vi "Settings Memory.vi"(6 "Write?":bool, 7 "Setting Choice":T2, 10 "Input":variant) -> (1 "PRL dt Tolerance":dbl, 2 "Output Int32":i32, 3 "Config Settings":T1)   [LabVIEW 2013, in "PMU Recorder Light.lvlib"]
uses:
  PMU Recorder Light.lvlib
  Configuration Settings.ctl
  Setting Choice.ctl
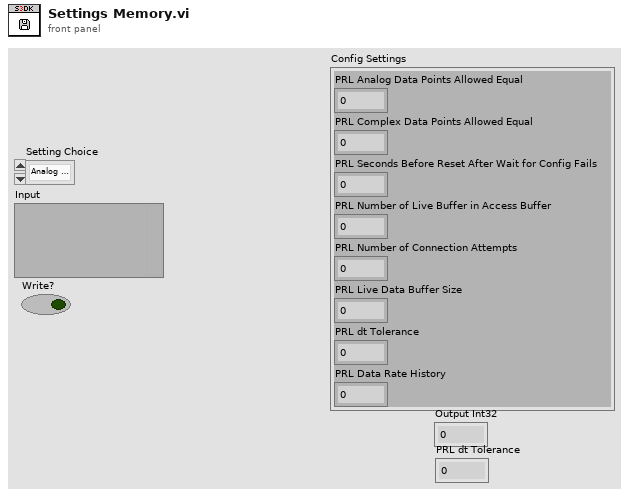
[diagram p1: front panel]
types:
  T1 = typedef "PMU Recorder Light.lvlib/Configuration Settings.ctl" = cluster{"PRL Analog Data Points Allowed Equal":i32, "PRL Complex Data Points Allowed Equal":i32, "PRL Seconds Before Reset After Wait for Config Fails":i32, "PRL Number of Live Buffer in Access Buffer":i32, "PRL Number of Connection Attempts":i32, "PRL Live Data Buffer Size":i32, "PRL dt Tolerance":dbl, "PRL Data Rate History":i32}
  T2 = typedef "PMU Recorder Light.lvlib/Setting Choice.ctl" = enum16{"Analog Data Points Allowed Equals", "Complex Data Points Allowed Equals", "Seconds Before Reset After Wait for Config Fails", "Number of Live Buffer in Access Buffer ", "Number of Connection Attempts", "Live Data Buffer Size", "dt Tolerance", "Data Rate History", "ALL"}
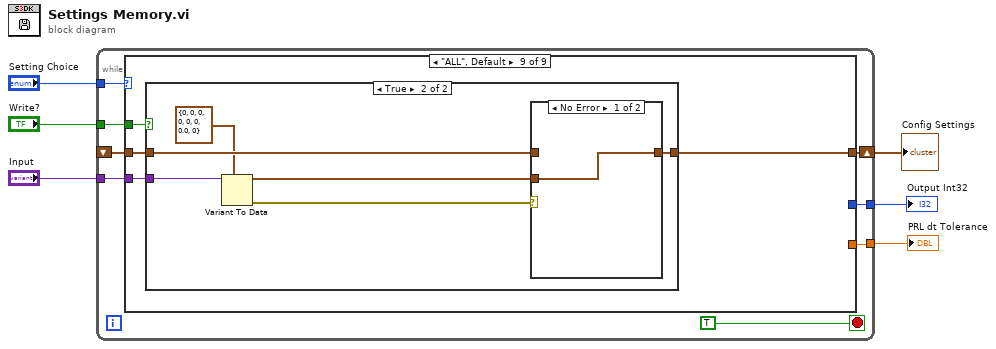
[diagram p0: block diagram]
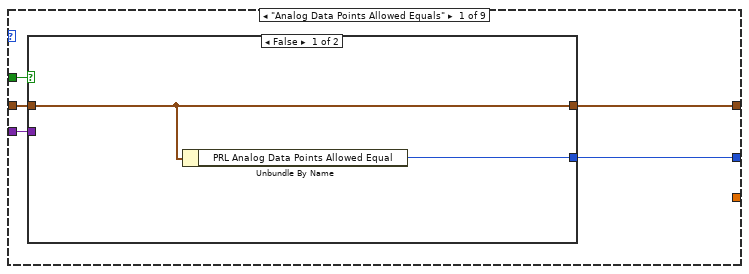
[diagram p2: hidden frame]
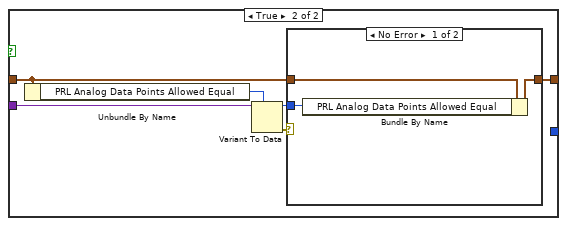
[diagram p3: hidden frame]
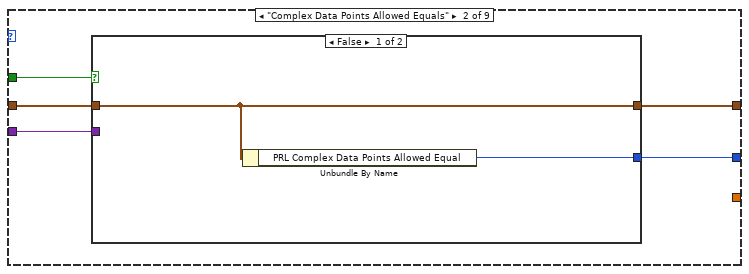
[diagram p5: hidden frame]
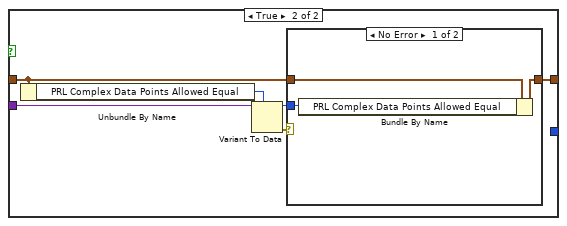
[diagram p6: hidden frame]
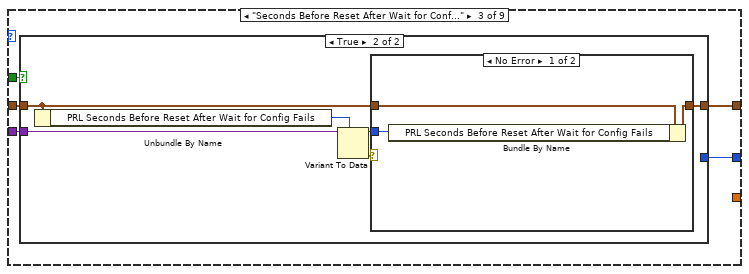
[diagram p8: hidden frame]
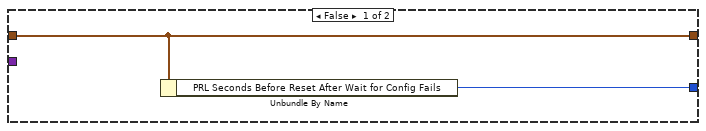
[diagram p9: hidden frame]
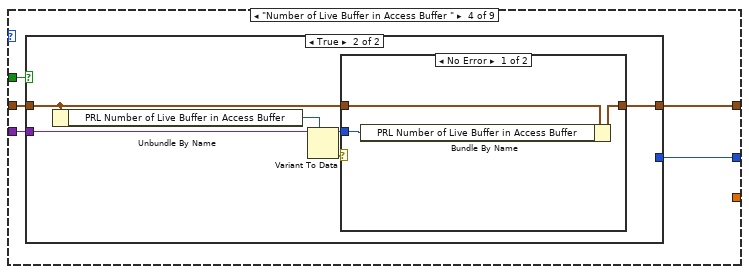
[diagram p11: hidden frame]
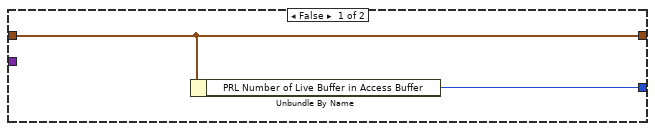
[diagram p12: hidden frame]
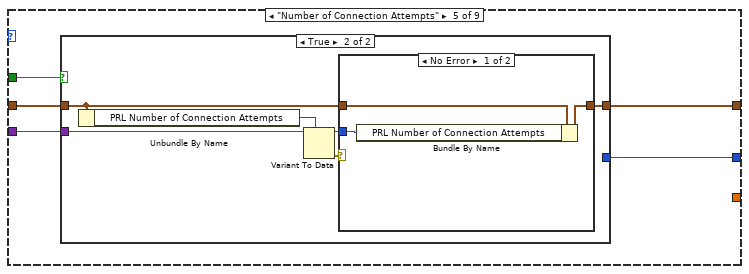
[diagram p14: hidden frame]
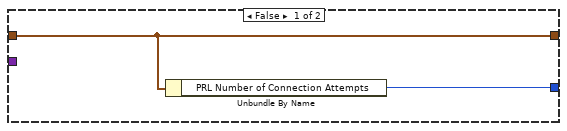
[diagram p15: hidden frame]
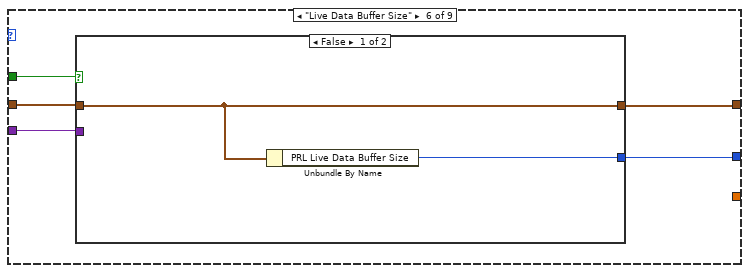
[diagram p17: hidden frame]
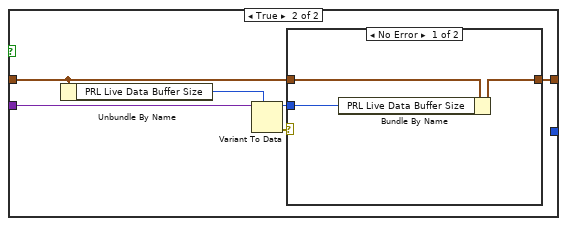
[diagram p18: hidden frame]
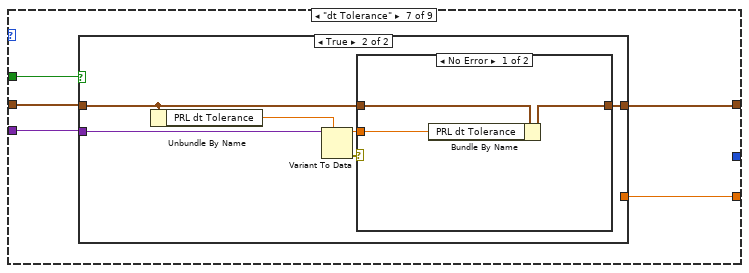
[diagram p20: hidden frame]
diagram:
  n1 = while {
    shift-right: [w13] -> w3
    shift-left: _ -> [w9]
    tunnel: "Setting Choice" -> [w14]
    tunnel: "Input" -> [w10]
    tunnel: "Write?" -> [w11]
    tunnel: [w8] -> w2
    tunnel: [w7] -> w1
    stop <- TRUE stop-if-true
    n2 = case shown="\"ALL\", Default" w14 {
      tunnel: w9 -> [w18 w34 w52 w70 w86 w103 w120 w137 w153]
      tunnel: [w16 w35 w49 w66 w84 w100 w118 w135 w154] -> w13
      tunnel: w11 -> [w17 w32 w53 w69 w87 w104 w121 w138 w152]
      tunnel: w10 -> [w19 w33 w51 w68 w85 w102 w119 w136 w151]
      tunnel: [w15 w36 w50 w67 w83 w101 _ w134 _] -> w8
      tunnel: [_ _ _ _ _ _ w117 _ _] -> w7
      frame "Analog Data Points Allowed Equals" {
        n3 = case shown="False" w17 {
          tunnel: [w21 w27] -> w16
          tunnel: w18 -> [w21 w23]
          tunnel: w19 -> [_ w26]
          tunnel: [w20 _] -> w15
          frame False {
            n4 = Unbundle By Name(w21) -> ("PRL Analog Data Points Allowed Equal"=w20:i32)
          }
          frame True {
            n5 = Unbundle By Name(w23) -> ("PRL Analog Data Points Allowed Equal"=w22:i32)
            n6 = Variant To Data(type=w22, Variant=w26) -> (data=w24:i32, error out=w25:errorcluster)  [unwired: 1 in]
            n7 = case shown="No Error" w25 {
              tunnel: [w28 w31] -> w27
              tunnel: w24 -> [w29 _]
              tunnel: w23 -> [w30 w31]
              frame No Error {
                n8 = Bundle By Name(cluster=w30, "PRL Analog Data Points Allowed Equal"=w29) -> (w28:T1)
              }
              frame Error {
              }
            }
          }
        }
      }
      frame "Complex Data Points Allowed Equals" {
        n9 = case shown="False" w32 {
          tunnel: [w38 w44] -> w35
          tunnel: w34 -> [w38 w40]
          tunnel: w33 -> [_ w43]
          tunnel: [w37 _] -> w36
          frame False {
            n10 = Unbundle By Name(w38) -> ("PRL Complex Data Points Allowed Equal"=w37:i32)
          }
          frame True {
            n11 = Unbundle By Name(w40) -> ("PRL Complex Data Points Allowed Equal"=w39:i32)
            n12 = Variant To Data(type=w39, Variant=w43) -> (data=w41:i32, error out=w42:errorcluster)  [unwired: 1 in]
            n13 = case shown="No Error" w42 {
              tunnel: [w45 w48] -> w44
              tunnel: w41 -> [w46 _]
              tunnel: w40 -> [w47 w48]
              frame No Error {
                n14 = Bundle By Name(cluster=w47, "PRL Complex Data Points Allowed Equal"=w46) -> (w45:T1)
              }
              frame Error {
              }
            }
          }
        }
      }
      frame "Seconds Before Reset After Wait for Config Fails" {
        n15 = case shown="True" w53 {
          tunnel: [w55 w61] -> w49
          tunnel: w52 -> [w55 w57]
          tunnel: w51 -> [_ w60]
          tunnel: [w54 _] -> w50
          frame False {
            n16 = Unbundle By Name(w55) -> ("PRL Seconds Before Reset After Wait for Config Fails"=w54:i32)
          }
          frame True {
            n17 = Unbundle By Name(w57) -> ("PRL Seconds Before Reset After Wait for Config Fails"=w56:i32)
            n18 = Variant To Data(type=w56, Variant=w60) -> (data=w58:i32, error out=w59:errorcluster)  [unwired: 1 in]
            n19 = case shown="No Error" w59 {
              tunnel: [w62 w65] -> w61
              tunnel: w58 -> [w63 _]
              tunnel: w57 -> [w64 w65]
              frame No Error {
                n20 = Bundle By Name(cluster=w64, "PRL Seconds Before Reset After Wait for Config Fails"=w63) -> (w62:T1)
              }
              frame Error {
              }
            }
          }
        }
      }
      frame "Number of Live Buffer in Access Buffer " {
        n21 = case shown="True" w69 {
          tunnel: [w72 w78] -> w66
          tunnel: w70 -> [w72 w74]
          tunnel: w68 -> [_ w77]
          tunnel: [w71 _] -> w67
          frame False {
            n22 = Unbundle By Name(w72) -> ("PRL Number of Live Buffer in Access Buffer"=w71:i32)
          }
          frame True {
            n23 = Unbundle By Name(w74) -> ("PRL Number of Live Buffer in Access Buffer"=w73:i32)
            n24 = Variant To Data(type=w73, Variant=w77) -> (data=w75:i32, error out=w76:errorcluster)  [unwired: 1 in]
            n25 = case shown="No Error" w76 {
              tunnel: [w79 w82] -> w78
              tunnel: w75 -> [w80 _]
              tunnel: w74 -> [w81 w82]
              frame No Error {
                n26 = Bundle By Name(cluster=w81, "PRL Number of Live Buffer in Access Buffer"=w80) -> (w79:T1)
              }
              frame Error {
              }
            }
          }
        }
      }
      frame "Number of Connection Attempts" {
        n27 = case shown="True" w87 {
          tunnel: [w89 w95] -> w84
          tunnel: w86 -> [w89 w91]
          tunnel: w85 -> [_ w94]
          tunnel: [w88 _] -> w83
          frame False {
            n28 = Unbundle By Name(w89) -> ("PRL Number of Connection Attempts"=w88:i32)
          }
          frame True {
            n29 = Unbundle By Name(w91) -> ("PRL Number of Connection Attempts"=w90:i32)
            n30 = Variant To Data(type=w90, Variant=w94) -> (data=w92:i32, error out=w93:errorcluster)  [unwired: 1 in]
            n31 = case shown="No Error" w93 {
              tunnel: [w96 w99] -> w95
              tunnel: w92 -> [w97 _]
              tunnel: w91 -> [w98 w99]
              frame No Error {
                n32 = Bundle By Name(cluster=w98, "PRL Number of Connection Attempts"=w97) -> (w96:T1)
              }
              frame Error {
              }
            }
          }
        }
      }
      frame "Live Data Buffer Size" {
        n33 = case shown="False" w104 {
          tunnel: [w106 w112] -> w100
          tunnel: w103 -> [w106 w108]
          tunnel: w102 -> [_ w111]
          tunnel: [w105 _] -> w101
          frame False {
            n34 = Unbundle By Name(w106) -> ("PRL Live Data Buffer Size"=w105:i32)
          }
          frame True {
            n35 = Unbundle By Name(w108) -> ("PRL Live Data Buffer Size"=w107:i32)
            n36 = Variant To Data(type=w107, Variant=w111) -> (data=w109:i32, error out=w110:errorcluster)  [unwired: 1 in]
            n37 = case shown="No Error" w110 {
              tunnel: [w113 w116] -> w112
              tunnel: w109 -> [w114 _]
              tunnel: w108 -> [w115 w116]
              frame No Error {
                n38 = Bundle By Name(cluster=w115, "PRL Live Data Buffer Size"=w114) -> (w113:T1)
              }
              frame Error {
              }
            }
          }
        }
      }
      frame "dt Tolerance" {
        n39 = case shown="True" w121 {
          tunnel: [w123 w129] -> w118
          tunnel: w120 -> [w123 w125]
          tunnel: w119 -> [_ w128]
          tunnel: [w122 _] -> w117
          frame False {
            n40 = Unbundle By Name(w123) -> ("PRL dt Tolerance"=w122:dbl)
          }
          frame True {
            n41 = Unbundle By Name(w125) -> ("PRL dt Tolerance"=w124:dbl)
            n42 = Variant To Data(type=w124, Variant=w128) -> (data=w126:dbl, error out=w127:errorcluster)  [unwired: 1 in]
            n43 = case shown="No Error" w127 {
              tunnel: [w130 w133] -> w129
              tunnel: w126 -> [w131 _]
              tunnel: w125 -> [w132 w133]
              frame No Error {
                n44 = Bundle By Name(cluster=w132, "PRL dt Tolerance"=w131) -> (w130:T1)
              }
              frame Error {
              }
            }
          }
        }
      }
      frame "Data Rate History" {
        n45 = case shown="True" w138 {
          tunnel: [w140 w146] -> w135
          tunnel: w137 -> [w140 w142]
          tunnel: w136 -> [_ w145]
          tunnel: [w139 _] -> w134
          frame False {
            n46 = Unbundle By Name(w140) -> ("PRL Data Rate History"=w139:i32)
          }
          frame True {
            n47 = Unbundle By Name(w142) -> ("PRL Data Rate History"=w141:i32)
            n48 = Variant To Data(type=w141, Variant=w145) -> (data=w143:i32, error out=w144:errorcluster)  [unwired: 1 in]
            n49 = case shown="No Error" w144 {
              tunnel: [w147 w150] -> w146
              tunnel: w143 -> [w148 _]
              tunnel: w142 -> [w149 w150]
              frame No Error {
                n50 = Bundle By Name(cluster=w149, "PRL Data Rate History"=w148) -> (w147:T1)
              }
              frame Error {
              }
            }
          }
        }
      }
      frame "ALL", Default {
        n51 = case shown="True" w152 {
          tunnel: [w155 w161] -> w154
          tunnel: w153 -> [w155 w157]
          tunnel: w151 -> [_ w160]
          frame False {
          }
          frame True {
            n52 = Variant To Data(type=T1 {"PRL Analog Data Points Allowed Equal"=0, "PRL Complex Data Points Allowed Equal"=0, "PRL Seconds Before Reset After Wait for Config Fails"=0, "PRL Number of Live Buffer in Access Buffer"=0, "PRL Number of Connection Attempts"=0, "PRL Live Data Buffer Size"=0, "PRL dt Tolerance"=0.0, "PRL Data Rate History"=0} ("Config Settings 2"), Variant=w160) -> (data=w158:T1, error out=w159:errorcluster)  [unwired: 1 in]
            n53 = case shown="No Error" w159 {
              tunnel: [w162 w163] -> w161
              tunnel: w158 -> [w162 _]
              tunnel: w157 -> [_ w163]
              frame No Error {
              }
              frame Error {
              }
            }
          }
        }
      }
    }
  }
  "Config Settings" <- w3
  "Output Int32" <- w2
  "PRL dt Tolerance" <- w1
